vi "Play_Rec_Data.vi"(8 "Zoom In Graph --->":dbl(slide)=0.573803 min=0.0 max=0.65 step=0.001 scale format="%#_1g", 9 "Play Speed":i32(knob)=1000 scale=100.0..2000.0, 10 "Stop Button":bool, 11 "Select path and filename":path) -> (3 "Recorded data":waveform(dbl)[](graph))   [LabVIEW 2012]
panel:
  out "EOF?":bool
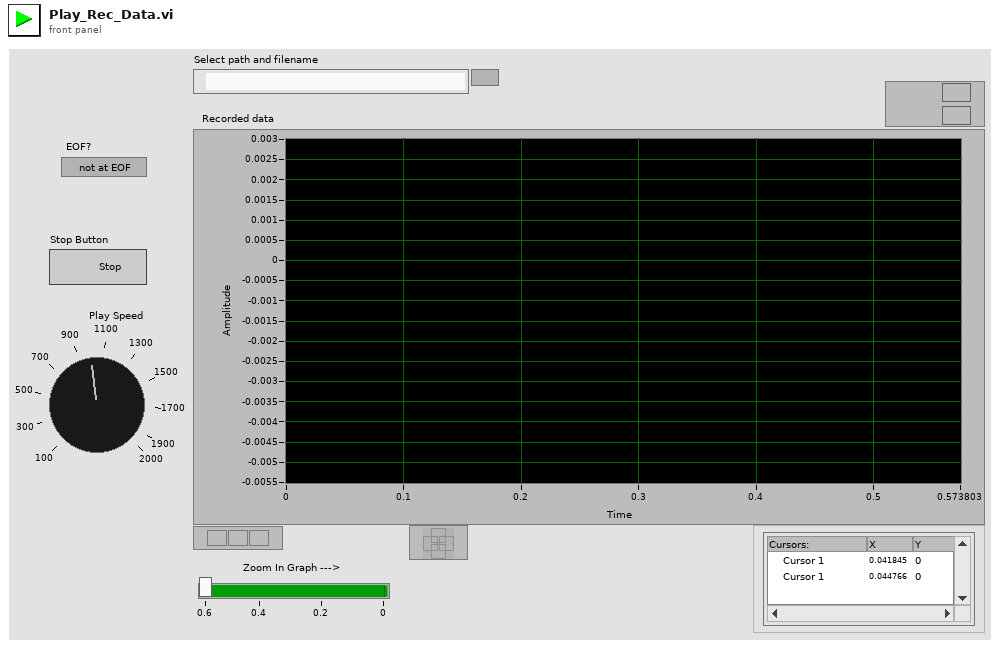
[diagram p1: front panel]
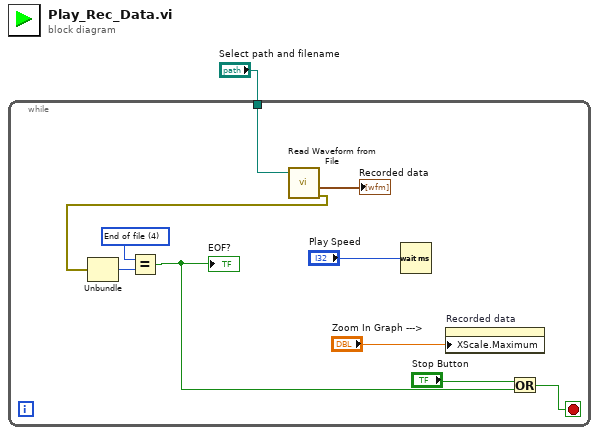
[diagram p0: block diagram]
diagram:
  n1 = while {
    tunnel: "Select path and filename" -> [w2]
    stop <- w3 stop-if-true
    w10 = 4 items=["No error", "Argument error", "Memory is full", "Out of zone", "End of file", "File already open", "Generic file I/O error", "File not found", "File permission error", "Disk is full", "Duplicate path", "Too many files open", "System feature not enabled", "Resource file not found", "Cannot add resource", "Resource not found", "Image not found", "Image memory error", "Pen does not exist", "Config type invalid", "Config token not found", "Config parse error", "Config memory error", "Bad external code format", "Bad external code offset", "External code not present", "Null window", "Destroy window error", "Null menu", "Print aborted", "Bad print record", "Print driver error", "Windows error during printing", "Memory error during printing", "Print dialog error", "Generic print error", "Invalid device refnum", "Device not found", "Device parameter error", "Device unit error", "Cannot open device", "Device call aborted", "Generic error", "Cancelled by user", "Object ID too low", "Object ID too high", "Object not in heap", "Unknown heap", "Unknown object (invalid DefProc)", "Unknown object (DefProc not in table)", "Message out of range", "Invalid (null) method", "Unknown message", "Manager call not supported", "Bad address", "Network operation in progress", "Network operation timed out", "Connection is busy", "Network attribute not supported", "Network error", "Address in use", "System out of memory", "Connection aborted", "Connection refused", "Not connected", "Already connected", "Connection closed", "Initialization error (interapplication manager)", "Bad occurrence", "Wait on unbound occurrence handler", "Occurrence queue overflow", "Datalog type conflict", "Unused", "Unrecognized type (interapplication manager)", "Memory corrupt", "Failed to make temporary DLL", "Old CIN version", "Unknown error code"]
    n2 = call <vilib>:"Read Waveform from File.vi"("file path (dialog if empty)"=w2) -> ("error out"=w8:errorcluster, "all waveforms in record"=→"Recorded data":waveform(dbl)[])  [unwired: 5 in, 2 out]
    n3 = Unbundle(w8) -> ("code"=w9:i32)  [unwired: 2 out]
    n4 = Equal?(x=w10, y=w9) -> (x = y?=w5:bool)
    "EOF?" <- w5
    n5 = Wait (ms)(milliseconds to wait="Play Speed") -> ()  [unwired: 1 out]
    n6 = property on="Recorded data" class="WFGraph (strict)"("XScale.Maximum"="Zoom In Graph --->") -> ()  [unwired: 2 in, 2 out]
    n7 = Or(x="Stop Button", y=w5) -> (x .or. y?=w3:bool)
  }
